vi "Query Many Registry.vi"(8 "error in":errorcluster, 11 "Name In":string[](array[string])) -> (0 "error out":errorcluster, 1 "Found":bool[](array[boolean]), 2 "Alias":string[](array[string]), 3 "Name Out":string[](array[string]))   [LabVIEW 2019, in "Identifier.lvclass"]
uses:
  Identifier.lvclass
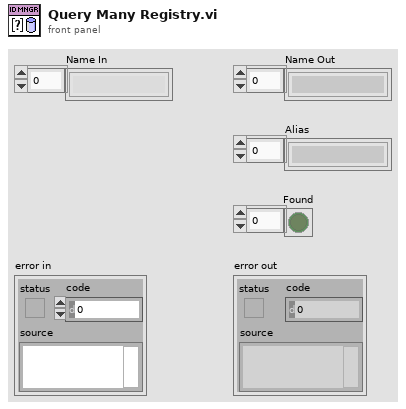
[diagram p1: front panel]
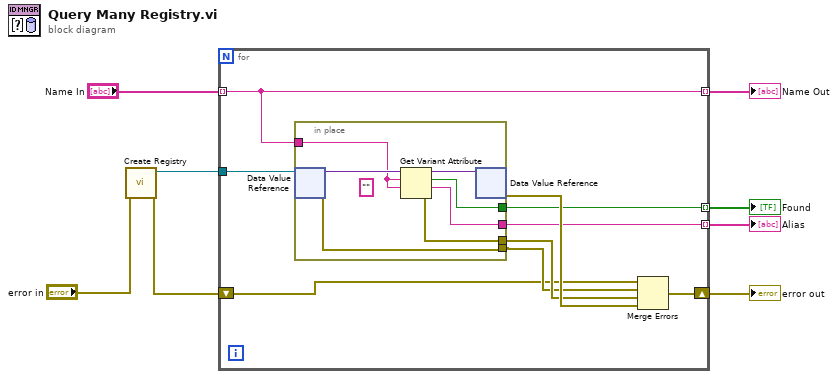
[diagram p0: block diagram]
diagram:
  n1 = call "Create Registry.vi"("error in"="error in") -> ("error out"=w2:errorcluster, "Registry"=w3:refnum<data-value>)  [unwired: 9 in]
  n2 = for {
    tunnel: "Name In" -> [w11] mode=indexing
    shift-right: [w14] -> w8
    shift-left: w2 -> [w9]
    tunnel: [w13] -> w6 mode=indexing
    tunnel: [w12] -> w5 mode=indexing
    tunnel: [w11] -> w4 mode=indexing
    tunnel: w3 -> [w10]
    n3 = in-place {
      in-place-border: w11 -> [w18]
      in-place-border: [w23] -> w12
      in-place-border: [w21] -> w13
      in-place-border: [w20] -> w15
      in-place-border: [w19] -> w16
      (unwired) ""
      n4 = in-place-dvr #1(w10) -> (w24:variant, w20:errorcluster)
      n5 = Get Variant Attribute(Variant=w24, name=w18, default value (empty Variant)=w18) -> (duplicate Variant=w22:variant, found=w21:bool, value=w23:string, error out=w19:errorcluster)  [unwired: 1 in]
      n6 = in-place-dvr #1(w22) -> (w17:errorcluster)  [unwired: 1 out]
    }
    n7 = Merge Errors(w9, w15, w16, w17) -> (w14:errorcluster)
  }
  "error out" <- w8
  "Alias" <- w5
  "Name Out" <- w4
  "Found" <- w6
